vi "test design tool.vi"() -> ()   [LabVIEW 2015, in "AguaClara Library.lvlib"]
uses:
  AguaClara Library.lvlib
  Project commands.ctl
  mathcad/Simple/MathCAD cmd.ctl
  AutoCAD cmds.ctl
  Project inputs.ctl
  User Information.ctl
  Basic Inputs.ctl
  Expert Inputs.ctl
  Variable cluster.ctl
  Country Ring.ctl
panel:
  in  "Set to Default":bool
  in  "Tab Control":enum32{"Page 1", "Page 2", "Page 3"}(tab)
  in  "Project inputs":T1={"Project Name"="junk", "City"="junk", "State"="", "Notes"=""}
  in  "User Information":T2={"First Name"="Monroe", "Last Name"="Weber-Shirk", "Email Address"="mw24@cornell.edu", "Organization"="enviro", "Language"=enum."English", "Country"=0} {"Country" items=["Afghanistan", "Aland Islands", "Albania", "Algeria", "American Samoa", "Andorra", "Angola", "Anguilla", "Antarctica", "Antigua And Barbuda", "Argentina", "Armenia", "Aruba", "Australia", "Austria", "Azerbaijan", "Bahamas", "Bahrain", "Bangladesh", "Barbados", "Belarus", "Belgium", "Belize", "Benin", "Bermuda", "Bhutan", "Bolivia", "Bosnia And Herzegovina", "Botswana", "Bouvet Island", "Brazil", "British Indian Ocean Territory", "Brunei Darussalam", "Bulgaria", "Burkina Faso", "Burundi", "Cambodia", "Cameroon", "Canada", "Cape Verde", "Cayman Islands", "Central African Republic", "Chad", "Chile", "China", "Christmas Island", "Cocos (Keeling) Islands", "Colombia", "Comoros", "Congo", "Congo, The Democratic Republic Of The", "Cook Islands", "Costa Rica", "Cote D'Ivoire", "Croatia", "Cuba", "Cyprus", "Czech Republic", "Denmark", "Djibouti", "Dominica", "Dominican Republic", "Ecuador", "Egypt", "El Salvador", "Equatorial Guinea", "Eritrea", "Estonia", "Ethiopia", "Falkland Islands (Malvinas)", "Faroe Islands", "Fiji", "Finland", "France", "French Guiana", "French Polynesia", "French Southern Territories", "Gabon", "Gambia", "Georgia", "Germany", "Ghana", "Gibraltar", "Greece", "Greenland", "Grenada", "Guadeloupe", "Guam", "Guatemala", "Guernsey", "Guinea", "Guinea-Bissau", "Guyana", "Haiti", "Heard Island And Mcdonald Islands", "Holy See (Vatican City State)", "Honduras", "Hong Kong", "Hungary", "Iceland", "India", "Indonesia", "Iran, Islamic Republic Of", "Iraq", "Ireland", "Isle Of Man", "Israel", "Italy", "Jamaica", "Japan", "Jersey", "Jordan", "Kazakhstan", "Kenya", "Kiribati", "Korea, Democratic People'S Republic Of", "Korea, Republic Of", "Kuwait", "Kyrgyzstan", "Lao People'S Democratic Republic", "Latvia", "Lebanon", "Lesotho", "Liberia", "Libyan Arab Jamahiriya", "Liechtenstein", "Lithuania", "Luxembourg", "Macao", "Macedonia, The Former Yugoslav Republic Of", "Madagascar", "Malawi", "Malaysia", "Maldives", "Mali", "Malta", "Marshall Islands", "Martinique", "Mauritania", "Mauritius", "Mayotte", "Mexico", "Micronesia, Federated States Of", "Moldova, Republic Of", "Monaco", "Mongolia", "Montserrat", "Morocco", "Mozambique", "Myanmar", "Namibia", "Nauru", "Nepal", "Netherlands", "Netherlands Antilles", "New Caledonia", "New Zealand", "Nicaragua", "Niger", "Nigeria", "Niue", "Norfolk Island", "Northern Mariana Islands", "Norway", "Oman", "Pakistan", "Palau", "Palestinian Territory, Occupied", "Panama", "Papua New Guinea", "Paraguay", "Peru", "Philippines", "Pitcairn", "Poland", "Portugal", "Puerto Rico", "Qatar", "Reunion", "Romania", "Russian Federation", "Rwanda", "Saint Helena", "Saint Kitts And Nevis", "Saint Lucia", "Saint Pierre And Miquelon", "Saint Vincent And The Grenadines", "Samoa", "San Marino", "Sao Tome And Principe", "Saudi Arabia", "Senegal", "Serbia And Montenegro", "Seychelles", "Sierra Leone", "Singapore", "Slovakia", "Slovenia", "Solomon Islands", "Somalia", "South Africa", "South Georgia And The South Sandwich Islands", "Spain", "Sri Lanka", "Sudan", "Suriname", "Svalbard And Jan Mayen", "Swaziland", "Sweden", "Switzerland", "Syrian Arab Republic", "Taiwan, Province Of China", "Tajikistan", "Tanzania, United Republic Of", "Thailand", "Timor-Leste", "Togo", "Tokelau", "Tonga", "Trinidad And Tobago", "Tunisia", "Turkey", "Turkmenistan", "Turks And Caicos Islands", "Tuvalu", "Uganda", "Ukraine", "United Arab Emirates", "United Kingdom", "United States", "United States Minor Outlying Islands", "Uruguay", "Uzbekistan", "Vanuatu", "Venezuela", "Viet Nam", "Virgin Islands, British", "Virgin Islands, U.S.", "Wallis And Futuna", "Western Sahara", "Yemen", "Zambia", "Zimbabwe", "(Not Specified)"]}
  in  "MathCAD results":T4
  out "error out":errorcluster
  in  "Design Inputs":T5={"Q.Plant"=0.005, "C.CoagDoseMax"=0.01, "C.CoagStock"=0.01, "Ti.CoagStock"=0.0015, "EN.DrillSeries"=enum."English", "EN.TubeSeries"=enum."English", "N.SedTanks"=10.0, "N.SedBaysEst"=120.0, "W.SedPlate"=0.01, "L.SedPlateSheet"=0.0, "T.SedPlate"=10031039.999999998, "T.PlantWall"=0.03, "H.FlocOption"=0.01, "T.FlocBaffleRigidH"=1.7999999999999998, "T.ConcreteMin"=0.3, "T.SedWeir"=0.04, "T.FlocBaffleRigidV"=108000.0} {"T.FlocBaffleRigidV" min=0.0 max=0.2 step=0.001 format="%#.1f"; "T.SedWeir" min=0.001 max=0.2 step=0.001 format="%#.1f"; "T.SedPlate" min=0.001 max=0.05 step=0.001 format="%#.1f"; "T.FlocBaffleRigidH" min=0.0 max=0.2 step=0.001 format="%#.1f"; "T.ConcreteMin" min=0.005 max=0.2 step=0.001 format="%#.1f"; "L.SedPlateSheet" min=0.3 max=8.0 step=0.01 format="%#.1f"; "N.SedBaysEst" min=1.0 max=20.0 step=1.0 format="%#.0f"; "N.SedTanks" min=1.0 max=20.0 step=1.0 format="%#.0f"; "Ti.CoagStock" min=43200.0 max=360000.0 step=3600.0 format="%#.1f"; "H.FlocOption" min=0.5 max=4.0 step=0.01 format="%#.2f"; "C.CoagStock" min=50.0 max=500.0 step=1.0 format="%#.0f"; "C.CoagDoseMax" min=0.03 max=0.2 step=0.005 format="%#.0f"; "Q.Plant" min=0.001 max=0.2 step=0.0001 format="%#.1f"; "T.PlantWall" min=0.05 max=0.5 step=0.001 format="%#.1f"; "W.SedPlate" min=0.5 max=3.0 step=0.001 format="%#.1f"}
  in  "Expert Inputs":T6={"V.EtUp"=0.001273148148148148, "ED.Rm"=0.0005, "W.FlocChannelMin"=0.45, "Pi.FlocBaffle"=45.0, "CP.Floc"=0.8, "ED.Floc"=[0.001, 0.0011, 0.002400000000000001], "ED.SedInlet"=0.01, "AN.SedManifoldBottom"=9.000000000000002e-07, "AN.SedManifoldTop"=0.08726646259971647, "Pi.FlowManifold"=59.99999999999999, "W.SedSludgeFlat"=0.008, "W.SedSludgeOverlap"=0.05, "Pi.FlowSludge"=5.0, "V.SedUpBod"=0.0008, "V.SedCBod"=0.0008101851851851852, "AN.SedPlate"=1.3395919067215362e-09, "S.SedPlateMin"=0.018277045187202513, "N.SedLaunders"=2.0, "Pi.FlowLaunder"=2.0, "HL.SedLaunderBod"=0.008, "B.SedLaunderOrifices"=0.05} {"N.SedLaunders" min=1.0 max=5.0 step=0.1 format="%#.1f"; "HL.SedLaunderBod" min=0.005 max=0.0098 step=0.0001 format="%#.2f"; "B.SedLaunderOrifices" min=0.02 max=0.1 step=0.001 format="%#.1f"; "Pi.FlowLaunder" min=1.0 max=4.0 step=1.0 format="%#.2f"; "W.SedSludgeOverlap" min=0.02 max=0.2 step=0.001 format="%#.1f"; "W.SedSludgeFlat" min=0.005 max=0.0098 step=0.0001 format="%#.2f"; "S.SedPlateMin" min=1.523087098933543 max=2.2846306484003143 step=0.0030461741978670856 format="%#.2f"; "AN.SedPlate" min=3.837648126251334e-08 max=2.3025888757508e-07 step=7.675296252502668e-09 format="%#.0f"; "AN.SedManifoldTop" min=0.0 max=0.3490658503988659 step=0.0017453292519943296 format="%#.2f"; "AN.SedManifoldBottom" min=5.729577951308232e-06 max=0.014323944878270581 step=5.729577951308232e-06 format="%#.1f"; "Pi.FlocBaffle" min=1.0 max=2.0 step=0.1 format="%#.2f"; "Pi.FlowSludge" min=2.0 max=20.0 step=0.1 format="%#.1f"; "ED.Rm" min=0.1 max=10.0 step=0.1 format="%#.1f"; "V.EtUp" min=0.005787037037037037 max=0.05787037037037037 step=0.0005787037037037037 format="%#.0f"; "V.SedCBod" min=0.0005787037037037037 max=0.0011574074074074073 step=1.1574074074074073e-05 format="%#.0f"; "V.SedUpBod" min=0.0005 max=0.00098 step=1e-05 format="%#.2f"; "Pi.FlowManifold" min=50.0 max=75.0 step=0.1 format="%#.2f"; "W.FlocChannelMin" min=0.1 max=2.0 step=0.001 format="%#.1f"; "ED.Floc" min=0.0001 max=0.25 step=0.0001 format="%#.1f"; "ED.SedInlet" min=0.001 max=0.005 step=0.0001 format="%#.2f"; "CP.Floc" min=30.0 max=300.0 step=1.0 format="%#.0f"}
  in  "AutoCAD Save":bool
  in  "AutoCAD Design":bool
  in  "Initialize CAD":bool
  out "got file paths":bool
  in  "Set File Paths":bool
  in  "Calculate":bool
  in  "Progress bar":dbl(slide) max=314.0 scale=0.0..1.0
  out "initialized CAD":bool
  in  "stop":bool
  in  "Send Design":bool
  in  "Save Design":bool
  in  "Get Values from MathCAD":bool
  in  "Send Expert Inputs to MathCAD":bool
  in  "Send Basic Inputs to MathCAD":bool
  in  "Create New Project":bool
  in  "Load User":bool
  # "save autocad file doesn't work yet"
  # "m^(2/3)"
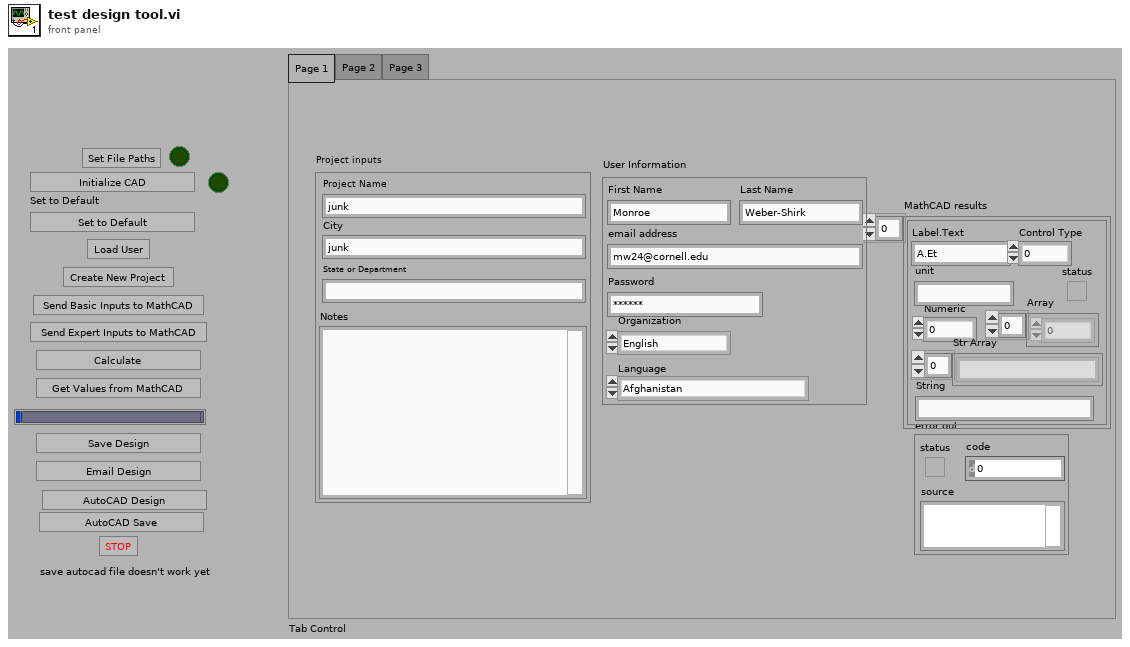
[diagram p1: front panel]
types:
  T1 = typedef "AguaClara Library.lvlib/Project inputs.ctl" = cluster{"Project Name":string, "City":string, "State":string, "Notes":string}
  T2 = typedef "AguaClara Library.lvlib/User Information.ctl" = cluster{"First Name":string, "Last Name":string, "Email Address":string, "Organization":string, "Language":enum16{"English", "Español", "French"}, "Country":T3}
  T3 = typedef "Country Ring.ctl" = u16
  T4 = typedef "Variable cluster.ctl" = cluster{"Label.Text":string, "Control Type":u32, "Numeric":dbl, "Array":dbl[], "status":bool, "Str Array":string[], "String":string, "unit":string}[]
  T5 = typedef "AguaClara Library.lvlib/Basic Inputs.ctl" = cluster{"Q.Plant":dbl[unit], "C.CoagDoseMax":dbl[unit], "C.CoagStock":dbl[unit], "Ti.CoagStock":dbl[unit], "EN.DrillSeries":enum16{"English", "Metric"}, "EN.TubeSeries":enum16{"English", "Metric"}, "N.SedTanks":dbl, "N.SedBaysEst":dbl, "W.SedPlate":dbl[unit], "L.SedPlateSheet":dbl[unit], "T.SedPlate":dbl[unit], "T.PlantWall":dbl[unit], "H.FlocOption":dbl[unit], "T.FlocBaffleRigidH":dbl[unit], "T.ConcreteMin":dbl[unit], "T.SedWeir":dbl[unit], "T.FlocBaffleRigidV":dbl[unit]}
  T6 = typedef "AguaClara Library.lvlib/Expert Inputs.ctl" = cluster{"V.EtUp":dbl[unit], "ED.Rm":dbl[unit], "W.FlocChannelMin":dbl[unit], "Pi.FlocBaffle":dbl, "CP.Floc":dbl, "ED.Floc":dbl[unit][], "ED.SedInlet":dbl[unit], "AN.SedManifoldBottom":dbl[unit], "AN.SedManifoldTop":dbl[unit], "Pi.FlowManifold":dbl, "W.SedSludgeFlat":dbl[unit], "W.SedSludgeOverlap":dbl[unit], "Pi.FlowSludge":dbl, "V.SedUpBod":dbl[unit], "V.SedCBod":dbl[unit], "AN.SedPlate":dbl[unit], "S.SedPlateMin":dbl[unit], "N.SedLaunders":dbl, "Pi.FlowLaunder":dbl, "HL.SedLaunderBod":dbl[unit], "B.SedLaunderOrifices":dbl[unit]}
  T7 = typedef "AguaClara Library.lvlib/Project commands.ctl" = enum16{"Load base file", "Load User", "Read paths", "Open Project", "New project", "Edit project", "Delete project", "Mail project", "save design", "open design"}
  T8 = typedef "MathCAD cmd.ctl" = enum16{"Open App", "Open Worksheet", "Close Worksheet", "Load Variable Ref", "Send Number", "Send Cluster", "Send Array", "Send String", "Calculate", "Get MathCAD data", "Close MathCAD"}
  T9 = typedef "AguaClara Library.lvlib/AutoCAD cmds.ctl" = enum16{"Open AutoCAD", "New Document", "Send Command", "Send Command Array", "Close Doc", "Quit"}
  T10 = typedef "Input Cluster.ctl" = cluster{"Project Info":T1, "Basic Inputs":T5}
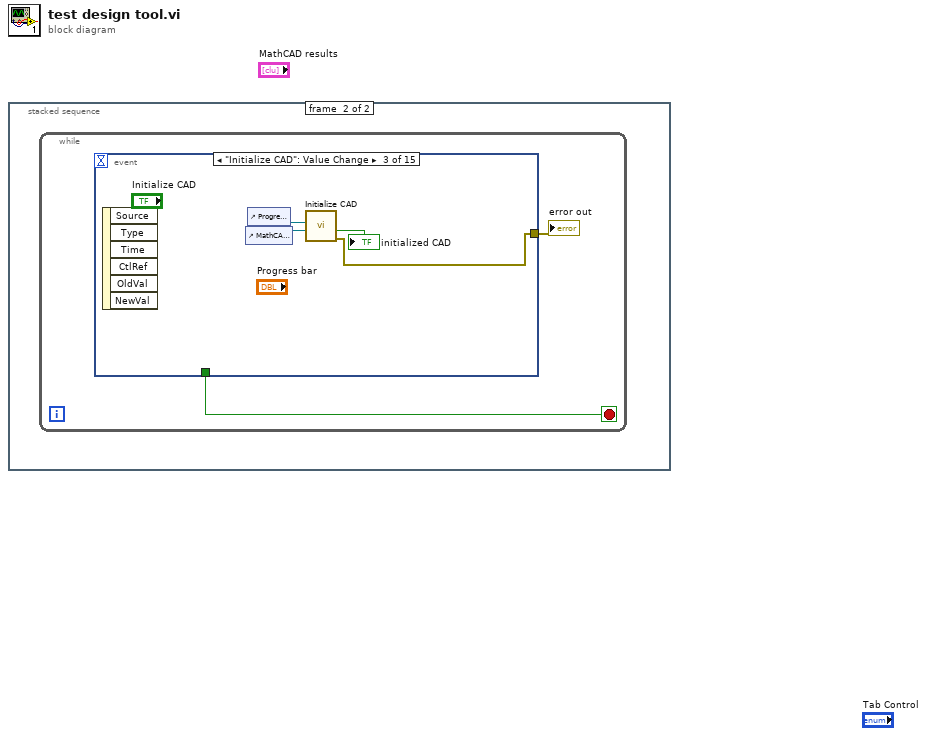
[diagram p0: block diagram]
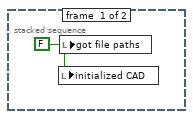
[diagram p2: hidden frame]
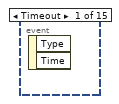
[diagram p3: hidden frame]
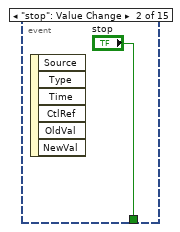
[diagram p4: hidden frame]
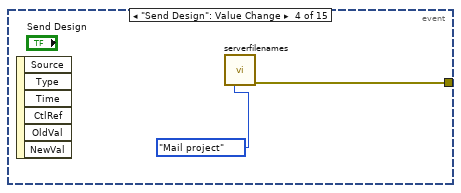
[diagram p5: hidden frame]
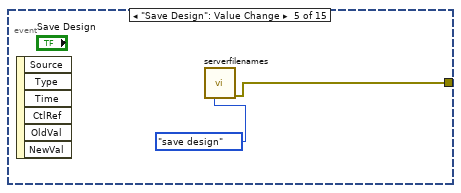
[diagram p6: hidden frame]
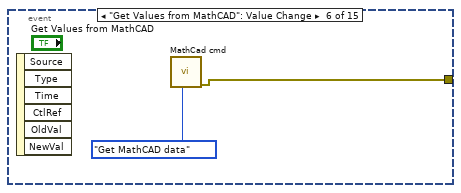
[diagram p7: hidden frame]
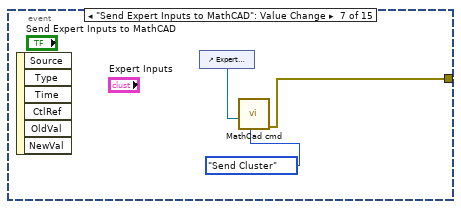
[diagram p8: hidden frame]
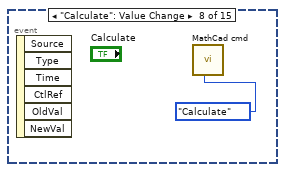
[diagram p9: hidden frame]
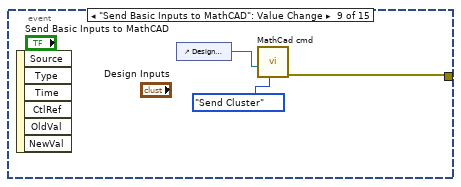
[diagram p10: hidden frame]
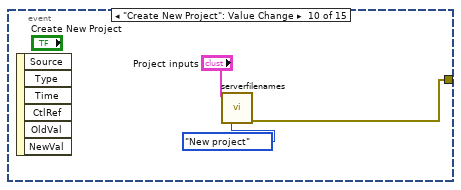
[diagram p11: hidden frame]
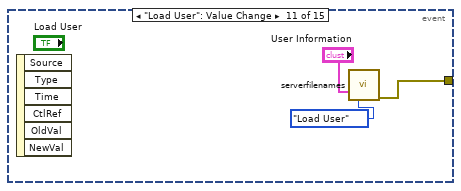
[diagram p12: hidden frame]
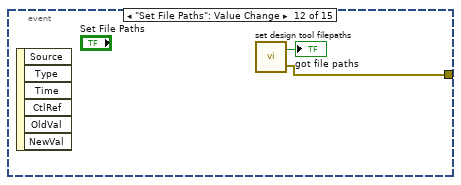
[diagram p13: hidden frame]
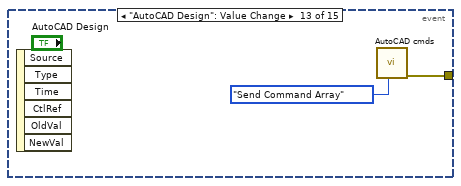
[diagram p14: hidden frame]
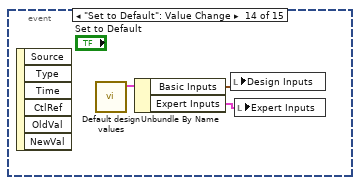
[diagram p15: hidden frame]
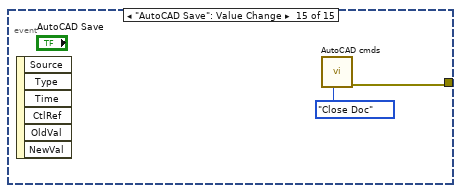
[diagram p16: hidden frame]
diagram:
  n1 = stacked-sequence {
    frame #0 {
      w1 = FALSE ("got file paths")
      n2 = local write "initialized CAD"(w1) -> ()
      n3 = local write "got file paths"(w1) -> ()
    }
    frame #1 {
      n4 = while {
        stop <- w3 stop-if-true
        n5 = event shown="[2] \"Initialize CAD\": Value Change" {
          selector: _ -> [_ _ _ _ _ _ _ _ _ _ _ _ _ _ _]
          dyn-events: _ -> [_ _ _ _ _ _ _ _ _ _ _ _ _ _ _]
          timeout: _ -> [_ _ _ _ _ _ _ _ _ _ _ _ _ _ _]
          tunnel: [_ "stop" _ _ _ _ _ _ _ _ _ _ _ _ _] -> w3
          tunnel: [_ _ w5 w9 w12 w13 w15 _ w19 w22 w25 w29 w30 _ w36] -> w2
          event Timeout {
            n6 = event-data() -> ()  [unwired: 1 in, 2 out]
          }
          event "stop": Value Change {
            n7 = event-data() -> ()  [unwired: 1 in, 6 out]
          }
          event "Initialize CAD": Value Change {
            n8 = event-data() -> ()  [unwired: 1 in, 6 out]
            n9 = control-ref of="MathCAD results"() -> (w8:refnum<vi>)
            n10 = control-ref of="Progress bar"() -> (w6:refnum<vi>)
            n11 = call "Initialize CAD.vi"(9:w8, 10:w6) -> ("error out"=w5:errorcluster, "Success"=→"initialized CAD":bool)  [unwired: 8 in]
          }
          event "Send Design": Value Change {
            n12 = event-data() -> ()  [unwired: 1 in, 6 out]
            n13 = call "serverfilenames.vi"("Project command"=Project_commands."Mail project") -> ("error out"=w9:errorcluster)  [unwired: 10 in, 4 out]
          }
          event "Save Design": Value Change {
            n14 = event-data() -> ()  [unwired: 1 in, 6 out]
            n15 = call "serverfilenames.vi"("Project command"=Project_commands."save design") -> ("error out"=w12:errorcluster)  [unwired: 10 in, 4 out]
          }
          event "Get Values from MathCAD": Value Change {
            n16 = event-data() -> ()  [unwired: 1 in, 6 out]
            n17 = call "MathCad cmd.vi"("MathCAD cmds"=MathCAD_cmd."Get MathCAD data") -> ("first error out"=w13:errorcluster)  [unwired: 9 in, 1 out]
          }
          event "Send Expert Inputs to MathCAD": Value Change {
            n18 = event-data() -> ()  [unwired: 1 in, 6 out]
            n19 = control-ref of="Expert Inputs"() -> (w17:refnum<vi>)
            n20 = call "MathCad cmd.vi"("MathCAD cmds"=MathCAD_cmd."Send Cluster", "Clust Refnum"=w17) -> ("first error out"=w15:errorcluster)  [unwired: 8 in, 1 out]
          }
          event "Calculate": Value Change {
            n21 = event-data() -> ()  [unwired: 1 in, 6 out]
            n22 = call "MathCad cmd.vi"("MathCAD cmds"=MathCAD_cmd."Calculate") -> ()  [unwired: 9 in, 2 out]
          }
          event "Send Basic Inputs to MathCAD": Value Change {
            n23 = event-data() -> ()  [unwired: 1 in, 6 out]
            n24 = control-ref of="Design Inputs"() -> (w20:refnum<vi>)
            n25 = call "MathCad cmd.vi"("MathCAD cmds"=MathCAD_cmd."Send Cluster", "Clust Refnum"=w20) -> ("first error out"=w19:errorcluster)  [unwired: 8 in, 1 out]
          }
          event "Create New Project": Value Change {
            n26 = event-data() -> ()  [unwired: 1 in, 6 out]
            n27 = call "serverfilenames.vi"("Project Info"="Project inputs", "Project command"=Project_commands."New project") -> ("error out"=w22:errorcluster)  [unwired: 9 in, 4 out]
          }
          event "Load User": Value Change {
            n28 = event-data() -> ()  [unwired: 1 in, 6 out]
            n29 = call "serverfilenames.vi"("User Information"="User Information", "Project command"=Project_commands."Load User") -> ("error out"=w25:errorcluster)  [unwired: 9 in, 4 out]
          }
          event "Set File Paths": Value Change {
            n30 = event-data() -> ()  [unwired: 1 in, 6 out]
            n31 = call "set design tool filepaths.vi"() -> ("error out"=w29:errorcluster, "Success"=→"got file paths":bool)  [unwired: 2 in]
          }
          event "AutoCAD Design": Value Change {
            n32 = event-data() -> ()  [unwired: 1 in, 6 out]
            n33 = call "AutoCAD cmds.vi"("AutoCAD cmd"=AutoCAD_cmds."Send Command Array") -> ("error out"=w30:errorcluster)  [unwired: 9 in, 1 out]
          }
          event "Set to Default": Value Change {
            n34 = event-data() -> ()  [unwired: 1 in, 6 out]
            n35 = call "Default design values.vi"() -> ("Input Cluster"=w34:T10)  [unwired: 9 in, 2 out]
            n36 = Unbundle By Name(w34) -> ("Basic Inputs"=w33:T5, "Expert Inputs"=w32:T6)
            n37 = local write "Design Inputs"(w33) -> ()
            n38 = local write "Expert Inputs"(w32) -> ()
          }
          event "AutoCAD Save": Value Change {
            n39 = event-data() -> ()  [unwired: 1 in, 6 out]
            n40 = call "AutoCAD cmds.vi"("AutoCAD cmd"=AutoCAD_cmds."Close Doc") -> ("error out"=w36:errorcluster)  [unwired: 9 in, 1 out]
          }
        }
        "error out" <- w2
      }
    }
  }
